vi "Create or get previous ref to image - pass calling vi ref for name.vi"(6 "Image Type":T2 items=["Grayscale (U8)", "Grayscale (I16)", "Grayscale (SGL)", "Complex (CSG)", "RGB (U32)", "HSL (U32)", "RGB (U64)", "Grayscale (U16)"], 8 "error in (no error)":errorcluster, 9 "Optional Name":string, 10 "Border Size":i32=5, 11 "Call VI ref":refnum<vi>) -> (0 "error out":errorcluster, 3 "Image":T1)   [LabVIEW 2013]
doc: "This vi (REENTRANT) will one the first call of each instance create an IMAQ image with the input boarder and input type using a name with the calling vi's label and optoinal string. Thereafter when called, it jst returns a reference from a shift register to the image."
uses:
  <vilib>/vision/Image Controls.llb/IMAQ Image.ctl
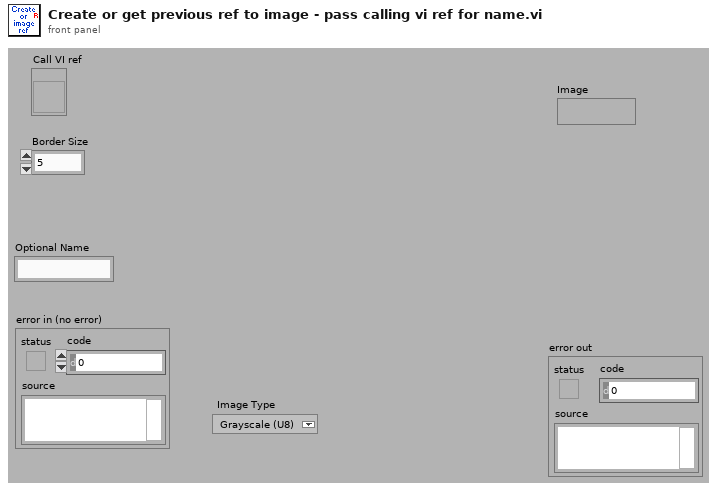
[diagram p1: front panel]
types:
  T1 = typedef "IMAQ Image.ctl" = refnum<image>
  T2 = typedef "Image Type" = u32
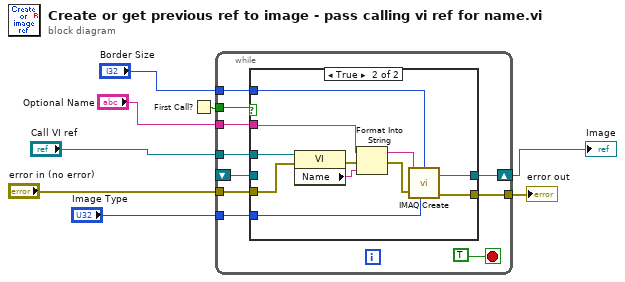
[diagram p0: block diagram]
diagram:
  n1 = First Call?() -> (First Call?: T/F=w4:bool)
  n2 = while {
    tunnel: [w18] -> w1
    tunnel: "error in (no error)" -> [w16]
    tunnel: w4 -> [w15]
    shift-right: [w17] -> w2
    shift-left: _ -> [w13]
    tunnel: "Call VI ref" -> [w12]
    tunnel: "Optional Name" -> [w11]
    tunnel: "Image Type" -> [w10]
    tunnel: "Border Size" -> [w9]
    stop <- TRUE ("stop") stop-if-true
    n3 = case shown="True" w15 {
      tunnel: [w19 w31] -> w18
      tunnel: [w20 w30] -> w17
      tunnel: w16 -> [w19 w24]
      tunnel: w13 -> [w20 _]
      tunnel: w12 -> [_ w27]
      tunnel: w11 -> [_ w21]
      tunnel: w10 -> [_ w23]
      tunnel: w9 -> [_ w22]
      frame False {
      }
      frame True {
        n4 = property class="VI"(reference=w27, error in=w24) -> (error out=w26:errorcluster, "Name"=w25:string)  [unwired: 1 out]
        n5 = Format Into String(initial string=w21, error in=w26, w25) -> (resulting string=w28:string, error out=w29:errorcluster)  [unwired: 1 in]
        n6 = call "IMAQ Create"("Border Size"=w22, "Image Name"=w28, "Image Type"=w23, "error in (no error)"=w29) -> ("New Image"=w30:T1, "error out"=w31:errorcluster)  [unwired: 1 out]
      }
    }
  }
  "Image" <- w2
  "error out" <- w1
